vi "TagSync.vi"() -> ()   [LabVIEW 2017]
uses:
  <vilib>/Utility/error.llb/DialogType.ctl
panel:
  in  "Sync Tagging":T1(tab)
  out "Minimum tagging period (pws)":u32=87
  out "Total tag data length (pws)":u32=86
  in  "TaggingPeriod (pws)":u32=155
  out "TagMarkerDuration (pws)":u16=10
  in  "PulseWidth (ms)":dbl=10.0
  out "Tag data does NOT fit in period!!!":bool
  in  "Halt tagging":bool
  in  "Calculate recommended tag settings":bool
  in  "Validate tag settings":bool
  out "Tag monitor":i16(graph)
  in  "Enable monitoring":bool
  out "Current tag number":i32=665
  out "Tag data":bool[](array[boolean])
  out "SyncTagOutput":bool
  in  "Minimum samples per pulse":dbl=10.0 format="%#_13g"
  in  "Minimum extra tag separation (pws)":u32=1
  in  "Minimum tags per file":u32=3
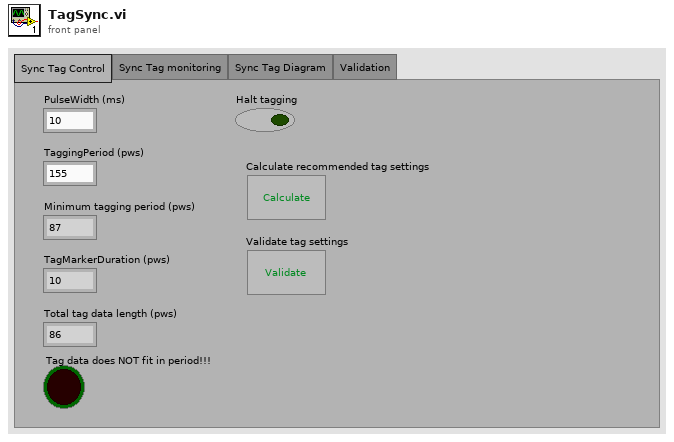
[diagram p1: front panel]
types:
  T1 = enum32{"Sync Tag Control", "Sync Tag monitoring", "Sync Tag Diagram", "Validation"}
  T2 = typedef "DialogType.ctl" = u16
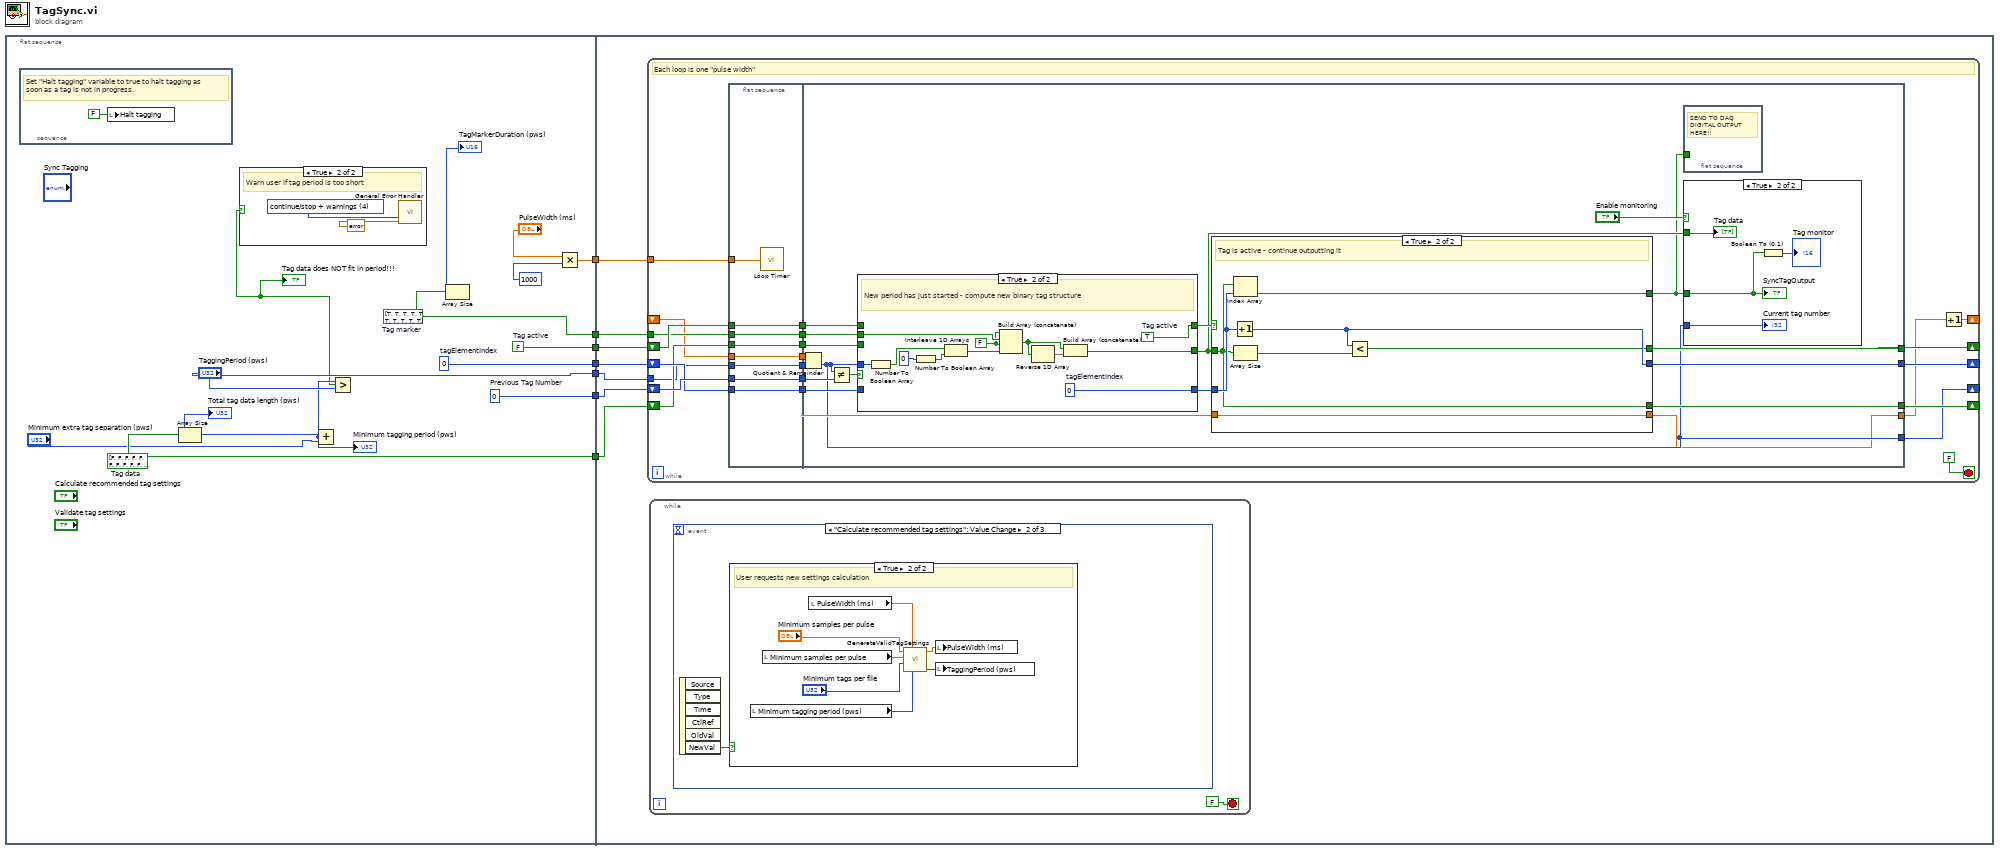
[diagram p0: block diagram]
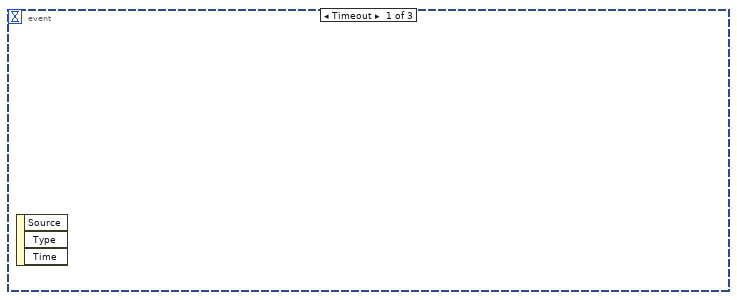
[diagram p3: hidden frame]
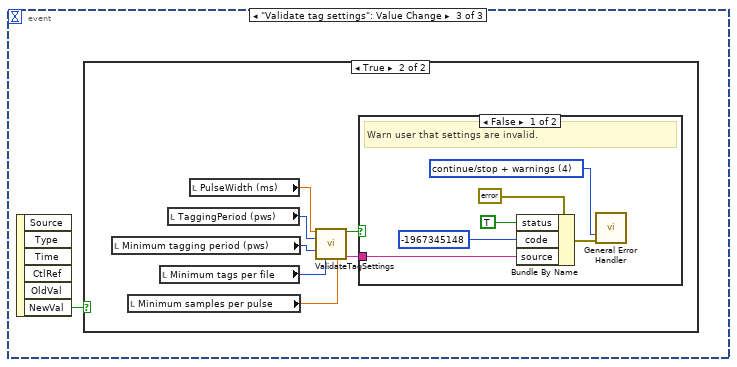
[diagram p5: hidden frame]
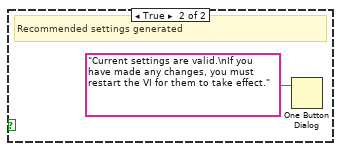
[diagram p7: hidden frame]
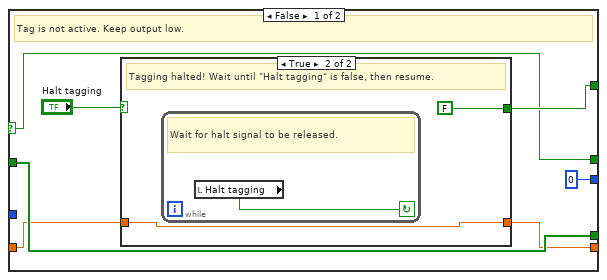
[diagram p9: hidden frame]
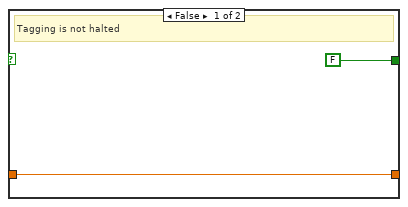
[diagram p10: hidden frame]
diagram:
  n1 = flat-sequence {
    tunnel: ["TaggingPeriod (pws)"] -> w7
    tunnel: [w14] -> w6
    tunnel: [w20] -> w5
    tunnel: [w19] -> w4
    tunnel: [w18] -> w3
    tunnel: [w17] -> w2
    tunnel: [w10] -> w1
    tunnel: w7 -> [w27]
    tunnel: w6 -> [w26]
    tunnel: w5 -> [w30]
    tunnel: w4 -> [w28]
    tunnel: w3 -> [w29]
    tunnel: w2 -> [w31]
    tunnel: w1 -> [w25]
    frame #0 {
      w14 = bool[] [TRUE, TRUE, TRUE, TRUE, TRUE, TRUE, TRUE, TRUE, TRUE, TRUE]  # Tag marker
      w19 = u32 0  # tagElementIndex
      w18 = FALSE  # Tag active
      w20 = bool[] [FALSE, FALSE, FALSE, FALSE, FALSE, FALSE, FALSE, FALSE, FALSE, FALSE, FALSE, FALSE, FALSE, FALSE, FALSE, FALSE, FALSE, FALSE, FALSE, FALSE, FALSE, FALSE, FALSE, FALSE, FALSE, FALSE, FALSE, FALSE, FALSE, FALSE, FALSE, FALSE, FALSE, FALSE, FALSE, FALSE, FALSE, FALSE, FALSE, FALSE, FALSE, FALSE, FALSE, FALSE, FALSE, FALSE, FALSE, FALSE, FALSE, FALSE, FALSE, FALSE, FALSE, FALSE, FALSE, FALSE, FALSE, FALSE, FALSE, FALSE, FALSE, FALSE, FALSE, FALSE, FALSE, FALSE, FALSE, FALSE, FALSE, FALSE, FALSE, FALSE, FALSE, FALSE, FALSE, FALSE, FALSE, FALSE, FALSE, FALSE, FALSE, FALSE, FALSE, FALSE, FALSE, FALSE, FALSE, FALSE, FALSE, FALSE, FALSE, FALSE, FALSE, FALSE, FALSE, FALSE, FALSE, FALSE, FALSE, FALSE, FALSE, FALSE, FALSE, FALSE, FALSE, FALSE, FALSE, FALSE, FALSE, FALSE, FALSE, FALSE, FALSE, FALSE, FALSE, FALSE, FALSE, FALSE, FALSE, FALSE, FALSE, FALSE, FALSE, FALSE, FALSE, FALSE, FALSE, FALSE, FALSE, FALSE, FALSE, FALSE, FALSE, FALSE, FALSE, FALSE, FALSE, FALSE, FALSE, FALSE, FALSE, FALSE, FALSE, FALSE, FALSE, FALSE, FALSE, FALSE, FALSE, FALSE, FALSE, FALSE]  # Tag data
      w17 = u32 0  # Previous Tag Number
      n2 = stacked-sequence {
        frame #0 {
          # "Set \"Halt tagging\" variable to true to halt tagging as soon as a tag is not in progress."
          n3 = local write "Halt tagging"(FALSE ("Halt tagging")) -> ()
        }
      }
      n4 = Array Size(array=w20) -> (size(s)=w9:i32)
      "Total tag data length (pws)" <- w9
      n5 = Add(x=w9, y="Minimum extra tag separation (pws)") -> (x+y=w15:u32)
      "Minimum tagging period (pws)" <- w15
      n6 = Greater?(x=w15, y="TaggingPeriod (pws)") -> (0:w13:bool)
      "Tag data does NOT fit in period!!!" <- w13
      n7 = case shown="True" w13 {
        frame False {
        }
        frame True {
          w22 = T2 4 items=["no dialog", "OK message", "continue or stop message", "OK message + warnings", "continue/stop + warnings"] ("type of dialog (OK msg:1)")
          # "Warn user if tag period is too short"
          n8 = call <vilib>:"General Error Handler.vi"("type of dialog (OK msg:1)"=w22, "error in (no error)"=errorcluster {"status"=TRUE, "code"=-1967345148, "source"="Warning! Tag data does not fit in period. \nPlease increase tag period and restart VI."}) -> ()  [unwired: 9 in, 5 out]
        }
      }
      n9 = Array Size(array=w14) -> (size(s)=→"TagMarkerDuration (pws)":i32)
      n10 = Multiply(x="PulseWidth (ms)", y=u32 1000) -> (x*y=w10:dbl)
    }
    frame #1 {
      n11 = while {
        shift-right: [w68] -> _
        shift-left: w31 -> [w77]
        shift-right: [w74] -> _
        shift-left: w30 -> [w71]
        shift-right: [w72] -> _
        shift-left: w29 -> [w76]
        shift-right: [w73] -> _
        shift-left: w28 -> [w75]
        tunnel: w27 -> [w70]
        tunnel: w26 -> [w69]
        tunnel: w25 -> [w61]
        shift-right: [w57] -> _
        shift-left: _ -> [w59]
        stop <- FALSE stop-if-true
        # "Each loop is one \"pulse width\""
        n12 = flat-sequence {
          tunnel: w69 -> [w80]
          tunnel: w70 -> [w81]
          tunnel: w71 -> [w82]
          tunnel: w75 -> [w83]
          tunnel: w76 -> [w84]
          tunnel: w77 -> [w85]
          tunnel: [w85] -> w67
          tunnel: [w84] -> w66
          tunnel: [w83] -> w65
          tunnel: [w82] -> w64
          tunnel: [w81] -> w63
          tunnel: [w80] -> w62
          tunnel: w61 -> [w78]
          tunnel: w59 -> [w79]
          tunnel: [w79] -> w58
          tunnel: w67 -> [w103]
          tunnel: w66 -> [w101]
          tunnel: w65 -> [w99]
          tunnel: w64 -> [w94]
          tunnel: w63 -> [w93]
          tunnel: w62 -> [w92]
          tunnel: w58 -> [w90]
          tunnel: [w97] -> w74
          tunnel: [w96] -> w73
          tunnel: [w95] -> w72
          tunnel: [w89] -> w68
          tunnel: [w88] -> w56
          frame #0 {
            n13 = call "Loop Timer"("Count(uSec)"=w78) -> ()  [unwired: 1 out]
          }
          frame #1 {
            n14 = Quotient & Remainder(x=w90, y=w93) -> (floor(x/y)=w89:u32)  [unwired: 1 out]
            n15 = Not Equal?(x=w89, y=w103) -> (x != y?=w102:bool)
            n16 = case shown="True" w102 {
              tunnel: w89 -> [_ w141]
              tunnel: w94 -> [w129 _]
              tunnel: w101 -> [w127 _]
              tunnel: [w127 w140] -> w100
              tunnel: [w129 w130] -> w91
              tunnel: w99 -> [w128 _]
              tunnel: [w128 w135] -> w98
              tunnel: w92 -> [_ w134]
              frame False {
              }
              frame True {
                w135 = u16 0  # tagElementIndex
                w133 = FALSE ("Marker on")
                w140 = TRUE  # Tag active
                # "New period has just started - compute new binary tag structure"
                n17 = Number To Boolean Array(number=w141) -> (Boolean array=w138:bool[])
                n18 = Number To Boolean Array(number=0) -> (Boolean array=w137:bool[])
                n19 = Interleave 1D Arrays(w138, w137) -> (w136:bool[])
                n20 = Build Array (concatenate)(w133, w134, w133, w136) -> (w131:bool[])
                n21 = Reverse 1D Array(array=w131) -> (reversed array=w132:bool[])
                n22 = Build Array (concatenate)(w131, w132) -> (w130:bool[])
              }
            }
            n23 = case shown="True" w100 {
              selector: w100 -> [w112 _]
              tunnel: w91 -> [w114 w123]
              tunnel: [w114 w123] -> w97
              tunnel: w98 -> [_ w126]
              tunnel: [u16 0 w122] -> w96
              tunnel: [w113 w125] -> w86
              tunnel: [w112 w121] -> w95
              tunnel: [w110 w120] -> w88
              tunnel: w90 -> [w109 w120]
              frame False {
                # "Tag is not active. Keep output low."
                n24 = case shown="True" "Halt tagging" {
                  tunnel: [FALSE ("Output 2") FALSE ("Output 2")] -> w113
                  tunnel: w109 -> [w116 w117]
                  tunnel: [w116 w117] -> w110
                  frame False {
                    # "Tagging is not halted"
                  }
                  frame True {
                    # "Tagging halted! Wait until \"Halt tagging\" is false, then resume."
                    n25 = while {
                      stop <- w119 continue-if-true
                      # "Wait for halt signal to be released."
                      n26 = local read "Halt tagging"() -> (w119:bool)
                    }
                  }
                }
              }
              frame True {
                # "Tag is active - continue outputting it"
                n27 = Increment(x=w126) -> (x+1=w122:u32)
                n28 = Index Array(array=w123, index=w126) -> (element=w125:bool)
                n29 = Array Size(array=w123) -> (size(s)=w124:i32)
                n30 = Less?(x=w122, y=w124) -> (x < y?=w121:bool)
              }
            }
            n31 = flat-sequence {
              tunnel: w86 -> [_]
              frame #0 {
                # "SEND TO DAQ DIGITAL OUTPUT HERE!!"
              }
            }
            n32 = case shown="True" "Enable monitoring" {
              tunnel: w91 -> [_ w107]
              tunnel: w86 -> [_ w104]
              tunnel: w89 -> [_ w105]
              frame False {
              }
              frame True {
                n33 = Boolean To (0,1)(Boolean=w104) -> (0, 1=→"Tag monitor":i16)
                "Current tag number" <- w105
                "Tag data" <- w107
                "SyncTagOutput" <- w104
              }
            }
          }
        }
        n34 = Increment(x=w56) -> (x+1=w57:dbl)
      }
      n35 = while {
        stop <- FALSE stop-if-true
        n36 = event shown="[1] \"Calculate recommended tag settings\": Value Change" {
          selector: _ -> [_ _ _]
          dyn-events: _ -> [_ _ _]
          timeout: _ -> [_ _ _]
          event Timeout {
            n37 = event-data() -> ()  [unwired: 1 in, 3 out]
          }
          event "Calculate recommended tag settings": Value Change {
            n38 = event-data() -> ("NewVal"=w33:bool)  [unwired: 1 in, 5 out]
            n39 = case shown="True" w33 {
              frame False {
              }
              frame True {
                # "User requests new settings calculation"
                n40 = local read "Minimum tagging period (pws)"() -> (w39:u32)
                n41 = local read "Minimum samples per pulse"() -> (w37:dbl)
                n42 = local read "PulseWidth (ms)"() -> (w35:dbl)
                n43 = call "GenerateValidTagSettings.vi"("Minimum tagging period (pws)"=w39, "PulseWidth (ms)"=w35, "Minimum tags per file"="Minimum tags per file", "Minimum samples per pulse"=w37, "Minimum samples per pulse 2"="Minimum samples per pulse") -> ("TaggingPeriod (pws)"=w34:u32, "lower limit"=w36:dbl)  [unwired: 5 in]
                n44 = local write "PulseWidth (ms)"(w36) -> ()
                n45 = local write "TaggingPeriod (pws)"(w34) -> ()
              }
            }
          }
          event "Validate tag settings": Value Change {
            n46 = event-data() -> ("NewVal"=w41:bool)  [unwired: 1 in, 5 out]
            n47 = case shown="True" w41 {
              frame False {
              }
              frame True {
                n48 = local read "Minimum tagging period (pws)"() -> (w48:u32)
                n49 = local read "Minimum samples per pulse"() -> (w47:dbl)
                n50 = local read "Minimum tags per file"() -> (w46:u32)
                n51 = local read "TaggingPeriod (pws)"() -> (w45:u32)
                n52 = local read "PulseWidth (ms)"() -> (w44:dbl)
                n53 = call "ValidateTagSettings.vi"("PulseWidth (ms)"=w44, "TaggingPeriod (pws)"=w45, "Minimum tagging period (pws)"=w48, "Minimum tags per file"=w46, "Minimum samples per pulse"=w47) -> ("Valid"=w43:bool, "Info"=w42:string)  [unwired: 9 in]
                n54 = case shown="False" w43 {
                  tunnel: w42 -> [w49 _]
                  frame False {
                    w54 = T2 4 items=["no dialog", "OK message", "continue or stop message", "OK message + warnings", "continue/stop + warnings"] ("type of dialog (OK msg:1)")
                    # "Warn user that settings are invalid."
                    n55 = Bundle By Name(cluster=errorcluster {"status"=FALSE, "code"=0, "source"=""} ("error in (no error)"), "status"=TRUE, "code"=-1967345148, "source"=w49) -> (w53:errorcluster)
                    n56 = call <vilib>:"General Error Handler.vi"("type of dialog (OK msg:1)"=w54, "error in (no error)"=w53) -> ()  [unwired: 9 in, 5 out]
                  }
                  frame True {
                    # "Recommended settings generated"
                    n57 = One Button Dialog(message="Current settings are valid.\nIf you have made any changes, you must restart the VI for them to take effect.") -> ()  [unwired: 1 in, 1 out]
                  }
                }
              }
            }
          }
        }
      }
    }
  }
